vi "Set DDS Out Mode.vi"(8 "error in (no error)":errorcluster, 10 "out_mode":u32, 11 "channel_index":u8) -> (0 "error out":errorcluster)   [LabVIEW 2021, in "vmmso.lvlib"]
doc: "DLL_API void WINAPI SetDDSOutMode(unsigned char channel_index, unsigned int out_mode);"
uses:
  vmmso.lvlib
  vmmso.dll
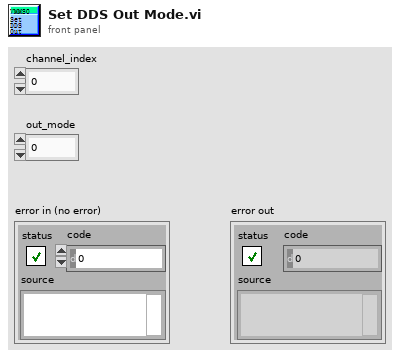
[diagram p1: front panel]
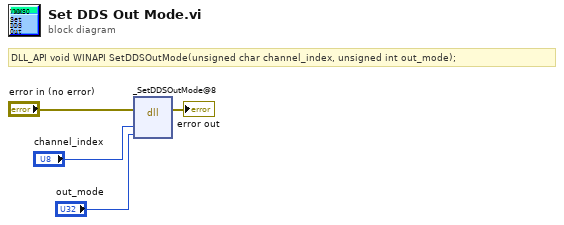
[diagram p0: block diagram]
diagram:
  # "DLL_API void WINAPI SetDDSOutMode(unsigned char channel_index, unsigned int out_mode);"
  n1 = dll-call lib="O:/MSO/library/demo-Labview/vmmso/vmmso.*" fn="_SetDDSOutMode@8"(error in="error in (no error)", "channel_index"="channel_index", "out_mode"="out_mode") -> (error out=→"error out":errorcluster)  [unwired: 5 in, 1 out]
